vi "Test Stack Operations.vi"() -> ()   [LabVIEW 2013]
uses:
  Circular Buffers/VariantBuffer/buffer-type -- enum.ctl
  <vilib>/addons/_JKI Toolkits/Caraya/classes/Assert/Assert True.vi
  Circular Buffers/VariantBuffer/VariantBuffer.lvclass
  <vilib>/addons/_JKI Toolkits/Caraya/classes/Test/Test.lvclass
  <vilib>/addons/_JKI Toolkits/Caraya/classes/Assert/Assert.lvclass
panel:
  out "elements 4":variant[](array[variant])
  out "error 548507":errorcluster
  out "elements 3":variant[](array[variant])
  out "elements 2":variant[](array[variant])
  out "elements":variant[](array[variant])
  out "error out 2":errorcluster
  out "error out":errorcluster
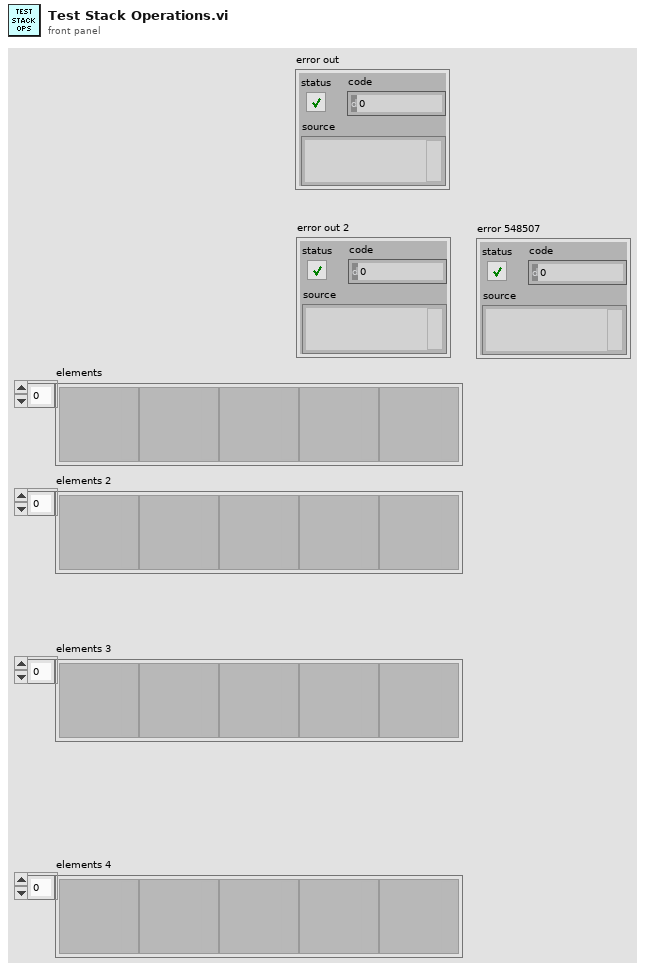
[diagram p1: front panel]
types:
  T1 = typedef "CircularBuffer.lvlib/VariantBuffer.lvclass/buffer-type -- enum.ctl" = enum16{"Queue", "Stack"}
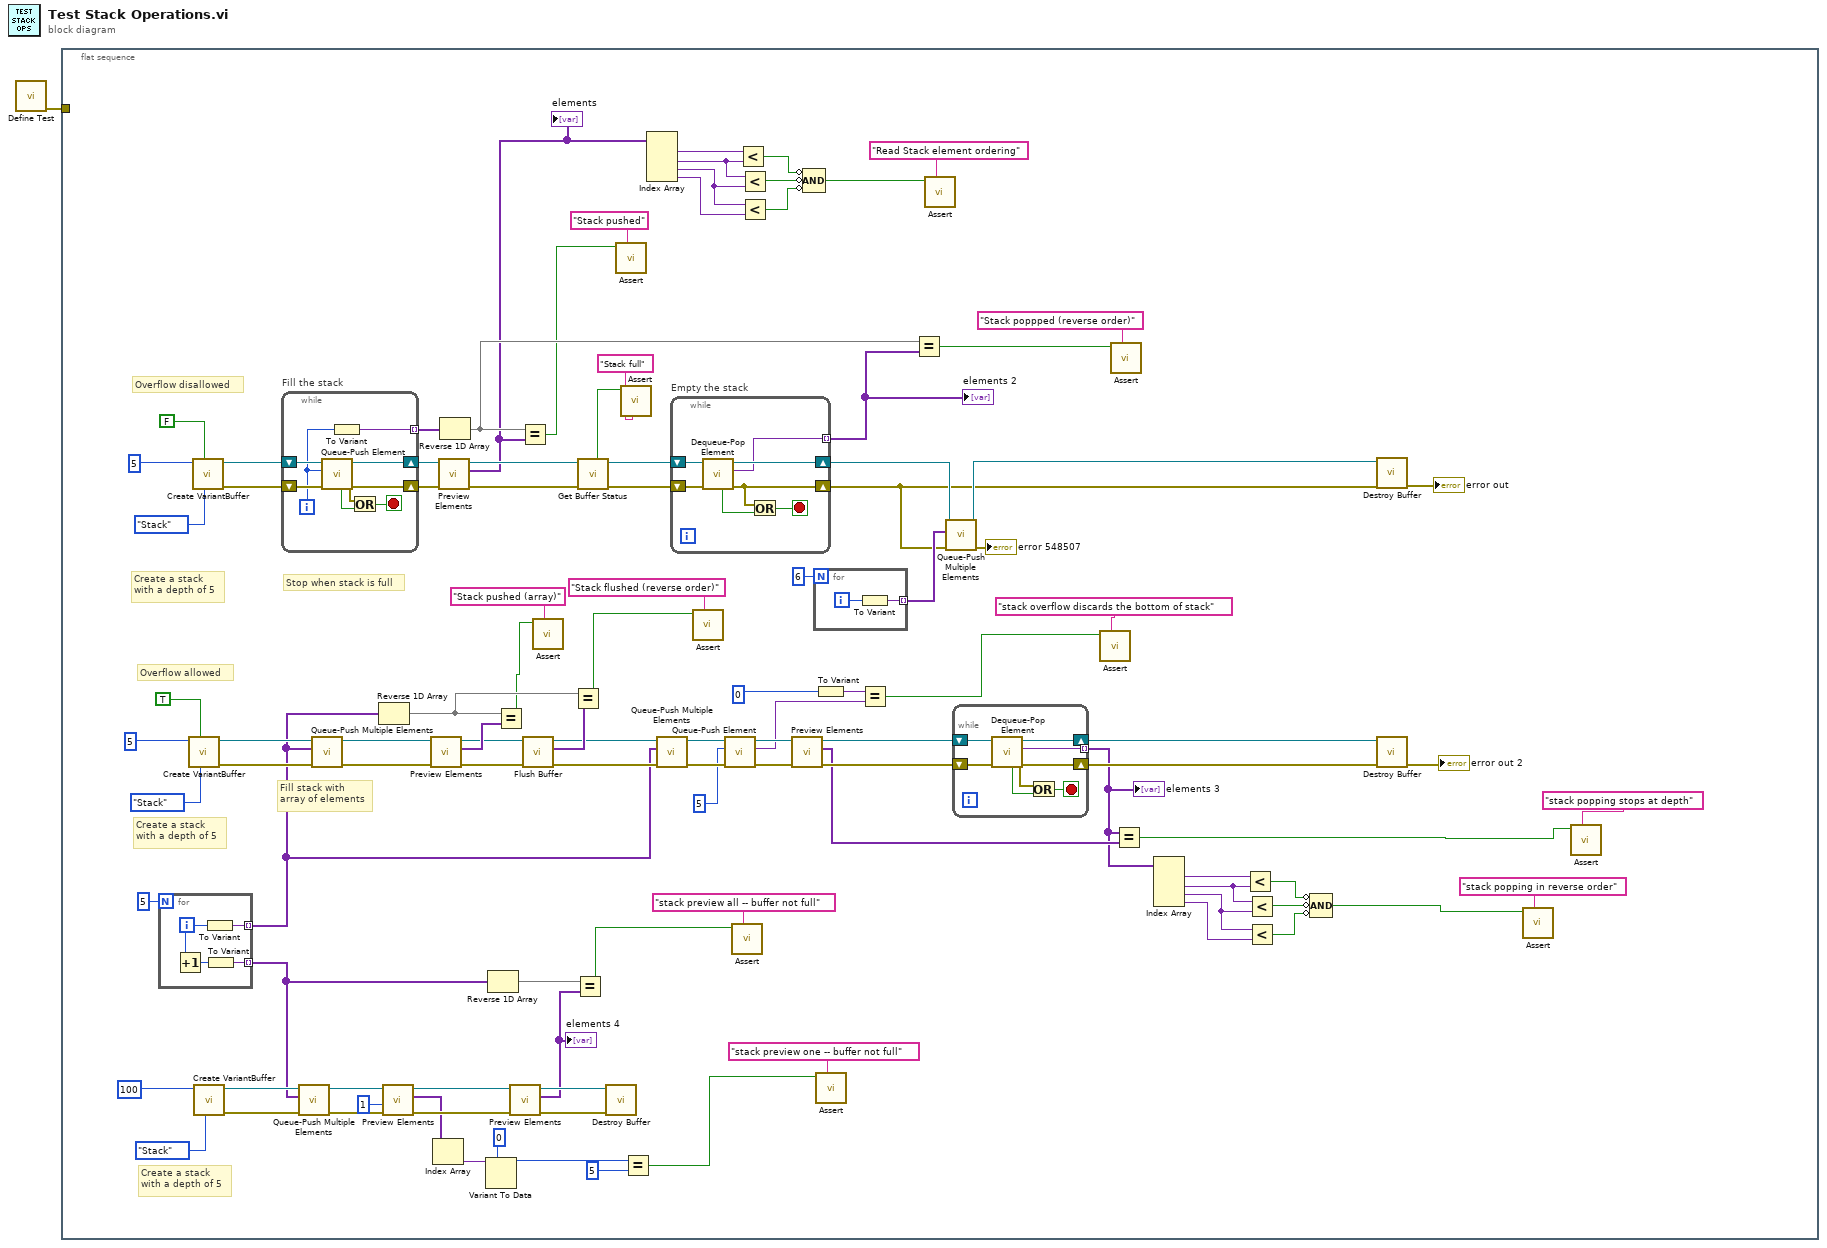
[diagram p0: block diagram]
diagram:
  n1 = call <vilib>:"Define Test.vi"() -> ("error out"=w1:errorcluster)  [unwired: 10 in, 1 out]
  n2 = flat-sequence {
    tunnel: w1 -> [_]
    frame #0 {
      # "Create a stack\nwith a depth of 5"
      # "Overflow disallowed"
      # "Overflow allowed"
      # "Fill stack with\narray of elements"
      # "Create a stack\nwith a depth of 5"
      # "Stop when stack is full"
      # "Create a stack\nwith a depth of 5"
      n3 = for {
        N: 5 -> [_]
        tunnel: [w122] -> w25 mode=indexing
        tunnel: [w119] -> w26 mode=indexing
        i -> [w120]
        n4 = Increment(x=w120) -> (x+1=w121:i32)
        n5 = To Variant(anything=w120) -> (Variant=w122:variant)
        n6 = To Variant(anything=w121) -> (Variant=w119:variant)
      }
      n7 = call "Create VariantBuffer.vi"("buffer-type"=buffer-type_--_enum."Stack", "Allow Overflow?"=TRUE ("Allow Overflow? (T)"), "bufSize"=5) -> ("error out"=w93:errorcluster, "Buffer"=w94:refnum<data-value>)  [unwired: 7 in]
      n8 = call "Create VariantBuffer.vi"("buffer-type"=buffer-type_--_enum."Stack", "Allow Overflow?"=FALSE ("Allow Overflow? (T)"), "bufSize"=5) -> ("error out"=w106:errorcluster, "Buffer"=w105:refnum<data-value>)  [unwired: 7 in]
      n9 = call "Create VariantBuffer.vi"("buffer-type"=buffer-type_--_enum."Stack", "bufSize"=100) -> ("error out"=w40:errorcluster, "Buffer"=w41:refnum<data-value>)  [unwired: 8 in]
      n10 = while "Fill the stack" {
        shift-right: [w130] -> w102
        shift-left: w106 -> [w137]
        shift-right: [w135] -> w103
        shift-left: w105 -> [w136]
        tunnel: [w133] -> w84 mode=indexing
        i -> [w134]
        stop <- w131 stop-if-true
        n11 = call "Queue-Push Element.vi"("error in"=w137, "element"=w134, "Buffer in"=w136) -> ("error out"=w130:errorcluster, "Buffer"=w135:refnum<data-value>, "full"=w132:bool)  [unwired: 4 in, 2 out]
        n12 = To Variant(anything=w134) -> (Variant=w133:variant)
        n13 = Or(x=w130, y=w132) -> (x .or. y?=w131:bool)
      }
      n14 = call "Queue-Push Multiple Elements.vi"("error in"=w40, "elements"=w26, "Buffer in"=w41) -> ("error out"=w34:errorcluster, "Buffer"=w36:refnum<data-value>)  [unwired: 6 in, 1 out]
      n15 = call "Queue-Push Multiple Elements.vi"("error in"=w93, "elements"=w25, "Buffer in"=w94) -> ("error out"=w90:errorcluster, "Buffer"=w91:refnum<data-value>)  [unwired: 6 in, 1 out]
      n16 = Reverse 1D Array(array=w25) -> (reversed array=w82:variant[])
      n17 = call "Preview Elements.vi"("error in"=w34, "count (-1: all)"=1, "ByteBuffer in"=w36) -> ("error out"=w33:errorcluster, "elements"=w30:variant[], "ByteBuffer"=w35:refnum<data-value>)  [unwired: 6 in]
      n18 = call "Preview Elements.vi"("error in"=w90, "ByteBuffer in"=w91) -> ("error out"=w87:errorcluster, "elements"=w89:variant[], "ByteBuffer"=w88:refnum<data-value>)  [unwired: 7 in]
      n19 = Index Array(array=w30) -> (element=w29:variant)  [unwired: 1 in]
      n20 = call "Preview Elements.vi"("error in"=w102, "ByteBuffer in"=w103) -> ("error out"=w99:errorcluster, "elements"=w74:variant[], "ByteBuffer"=w101:refnum<data-value>)  [unwired: 7 in]
      "elements" <- w74
      n21 = Reverse 1D Array(array=w84) -> (reversed array=w83:variant[])
      n22 = Variant To Data(type=0 ("count (-1: all)"), Variant=w29) -> (data=w28:i32)  [unwired: 1 in, 1 out]
      n23 = Reverse 1D Array(array=w26) -> (reversed array=w24:variant[])
      n24 = Equal?(x=w82, y=w89) -> (x = y?=w14:bool)
      n25 = call "Preview Elements.vi"("error in"=w33, "ByteBuffer in"=w35) -> ("error out"=w38:errorcluster, "elements"=w32:variant[], "ByteBuffer"=w39:refnum<data-value>)  [unwired: 7 in]
      "elements 4" <- w32
      n26 = Equal?(x=w83, y=w74) -> (x = y?=w19:bool)
      n27 = call "Flush Buffer.vi"("error in"=w87, "Buffer in"=w88) -> ("error out"=w71:errorcluster, "elements"=w86:variant[], "Buffer"=w72:refnum<data-value>)  [unwired: 7 in]
      n28 = call-poly <vilib>:"Assert.vi"("Label"="Stack pushed (array)", "True?"=w14) -> ()  [unwired: 8 in, 2 out]
      n29 = Equal?(x=w82, y=w86) -> (x = y?=w13:bool)
      n30 = Equal?(x=w24, y=w32) -> (x = y?=w3:bool)
      n31 = call "Get Buffer Status.vi"("error in"=w99, "Buffer in"=w101) -> ("error out"=w98:errorcluster, "Buffer"=w100:refnum<data-value>, "full"=w20:bool)  [unwired: 5 in, 2 out]
      n32 = call "Destroy Buffer.vi"("error in"=w38, "Buffer"=w39) -> ()  [unwired: 8 in, 2 out]
      n33 = call-poly <vilib>:"Assert.vi"("Label"="Stack pushed", "True?"=w19) -> ()  [unwired: 8 in, 2 out]
      n34 = call-poly <vilib>:"Assert.vi"("Label"="Stack full", "True?"=w20) -> ()  [unwired: 8 in, 2 out]
      n35 = Equal?(x=w28, y=5 ("count (-1: all)")) -> (x = y?=w2:bool)
      n36 = Index Array(array=w74) -> (element #1=w81:variant, element #2=w80:variant, element #3=w79:variant, element #4=w78:variant)  [unwired: 4 in]
      n37 = call "Queue-Push Multiple Elements.vi"("error in"=w71, "elements"=w25, "Buffer in"=w72) -> ("error out"=w69:errorcluster, "Buffer"=w70:refnum<data-value>)  [unwired: 6 in, 1 out]
      n38 = while "Empty the stack" {
        shift-right: [w127] -> w49
        shift-left: w100 -> [w129]
        shift-right: [w126] -> w44
        shift-left: w98 -> [w128]
        tunnel: [w124] -> w73 mode=indexing
        stop <- w125 stop-if-true
        n39 = call "Dequeue-Pop Element.vi"("error in"=w128, "Buffer in"=w129) -> ("error out"=w126:errorcluster, "element"=w124:variant, "Buffer"=w127:refnum<data-value>, "buffer empty?"=w123:bool)  [unwired: 5 in, 1 out]
        n40 = Or(x=w126, y=w123) -> (x .or. y?=w125:bool)
      }
      "elements 2" <- w73
      n41 = call-poly <vilib>:"Assert.vi"("Label"="Stack flushed (reverse order)", "True?"=w13) -> ()  [unwired: 8 in, 2 out]
      n42 = call "Queue-Push Element.vi"("error in"=w69, "element"=5, "Buffer in"=w70) -> ("error out"=w66:errorcluster, "overflow"=w65:variant, "Buffer"=w67:refnum<data-value>)  [unwired: 4 in, 2 out]
      n43 = call-poly <vilib>:"Assert.vi"("Label"="stack preview all -- buffer not full", "True?"=w3) -> ()  [unwired: 8 in, 2 out]
      n44 = Less?(x=w81, y=w80) -> (x < y?=w75:bool)
      n45 = Less?(x=w80, y=w79) -> (x < y?=w77:bool)
      n46 = Less?(x=w79, y=w78) -> (x < y?=w76:bool)
      n47 = call "Preview Elements.vi"("error in"=w66, "ByteBuffer in"=w67) -> ("error out"=w60:errorcluster, "elements"=w58:variant[], "ByteBuffer"=w62:refnum<data-value>)  [unwired: 7 in]
      n48 = Compound Arithmetic op=AND(invert w75, invert w77, invert w76) -> (w23:bool)
      n49 = for {
        N: 6 -> [_]
        tunnel: [w110] -> w47 mode=indexing
        i -> [w111]
        n50 = To Variant(anything=w111) -> (Variant=w110:variant)
      }
      n51 = To Variant(anything=0) -> (Variant=w63:variant)
      n52 = call-poly <vilib>:"Assert.vi"("Label"="stack preview one -- buffer not full", "True?"=w2) -> ()  [unwired: 8 in, 2 out]
      n53 = Equal?(x=w63, y=w65) -> (x = y?=w10:bool)
      n54 = Equal?(x=w83, y=w73) -> (x = y?=w16:bool)
      n55 = call-poly <vilib>:"Assert.vi"("Label"="Read Stack element ordering", "True?"=w23) -> ()  [unwired: 8 in, 2 out]
      n56 = call "Queue-Push Multiple Elements.vi"("error in"=w44, "elements"=w47, "Buffer in"=w49) -> ("error out"=→"error 548507":errorcluster, "Buffer"=w45:refnum<data-value>)  [unwired: 6 in, 1 out]
      n57 = while {
        shift-right: [w117] -> w61
        shift-left: w62 -> [w118]
        shift-right: [w114] -> w59
        shift-left: w60 -> [w116]
        tunnel: [w113] -> w50 mode=indexing
        stop <- w115 stop-if-true
        n58 = call "Dequeue-Pop Element.vi"("error in"=w116, "Buffer in"=w118) -> ("error out"=w114:errorcluster, "element"=w113:variant, "Buffer"=w117:refnum<data-value>, "buffer empty?"=w112:bool)  [unwired: 5 in, 1 out]
        n59 = Or(x=w114, y=w112) -> (x .or. y?=w115:bool)
      }
      "elements 3" <- w50
      n60 = call-poly <vilib>:"Assert.vi"("Label"="stack overflow discards the bottom of stack", "True?"=w10) -> ()  [unwired: 8 in, 2 out]
      n61 = call-poly <vilib>:"Assert.vi"("Label"="Stack poppped (reverse order)", "True?"=w16) -> ()  [unwired: 8 in, 2 out]
      n62 = Equal?(x=w50, y=w58) -> (x = y?=w8:bool)
      n63 = Index Array(array=w50) -> (element #1=w51:variant, element #2=w52:variant, element #3=w53:variant, element #4=w54:variant)  [unwired: 4 in]
      n64 = Less?(x=w51, y=w52) -> (x < y?=w57:bool)
      n65 = Less?(x=w52, y=w53) -> (x < y?=w55:bool)
      n66 = Less?(x=w53, y=w54) -> (x < y?=w56:bool)
      n67 = Compound Arithmetic op=AND(invert w57, invert w55, invert w56) -> (w7:bool)
      n68 = call "Destroy Buffer.vi"("error in"=w44, "Buffer"=w45) -> ("error out"=→"error out":errorcluster)  [unwired: 8 in, 1 out]
      n69 = call "Destroy Buffer.vi"("error in"=w59, "Buffer"=w61) -> ("error out"=→"error out 2":errorcluster)  [unwired: 8 in, 1 out]
      n70 = call-poly <vilib>:"Assert.vi"("Label"="stack popping in reverse order", "True?"=w7) -> ()  [unwired: 8 in, 2 out]
      n71 = call-poly <vilib>:"Assert.vi"("Label"="stack popping stops at depth", "True?"=w8) -> ()  [unwired: 8 in, 2 out]
    }
  }
